vi "rethinkdb_launch.vi"(8 "error in (no error)":errorcluster, 9 "data_dir (\"\"=<appdir>\\rethinkdb_data)":path, 10 "http-port (5001)":u16=5001, 11 "rethinkdb.exe (\"\"=<appdir>\\rethinkdb.exe)":path) -> (0 "error out":errorcluster)   [LabVIEW 2017]
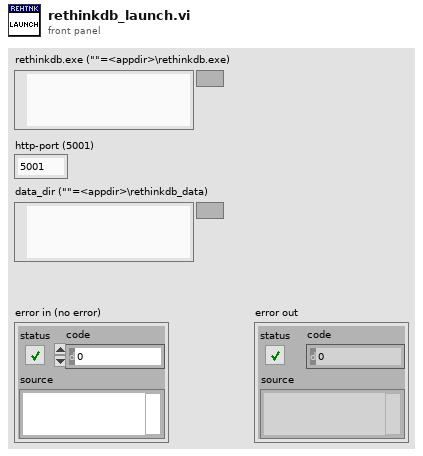
[diagram p1: front panel]
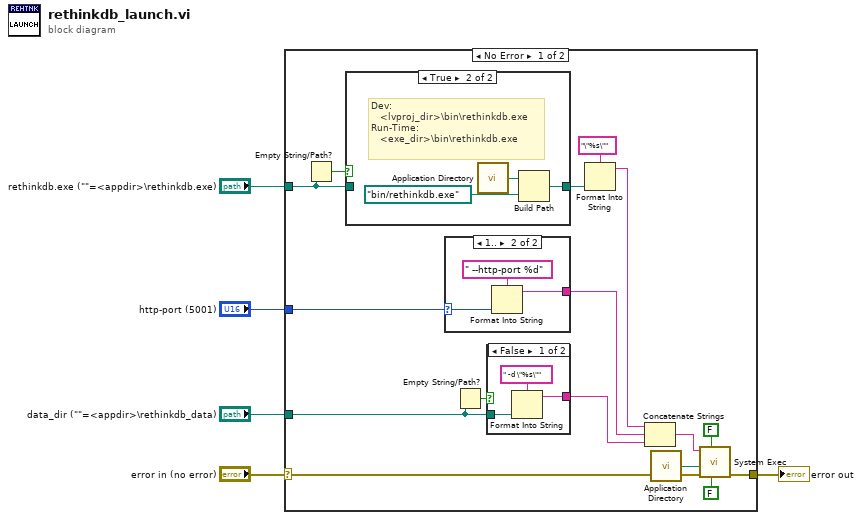
[diagram p0: block diagram]
diagram:
  n1 = case shown="No Error" "error in (no error)" {
    selector: "error in (no error)" -> [w21 w32]
    tunnel: [w20 w32] -> w4
    tunnel: "rethinkdb.exe (\"\"=<appdir>\\rethinkdb.exe)" -> [w16 _]
    tunnel: "http-port (5001)" -> [w14 _]
    tunnel: "data_dir (\"\"=<appdir>\\rethinkdb_data)" -> [w11 _]
    frame No Error {
      n2 = Empty String/Path?(string/path=w16) -> (empty?=w15:bool)
      n3 = case shown="True" w15 {
        tunnel: [w25 w27] -> w18
        tunnel: w16 -> [w25 _]
        frame False {
        }
        frame True {
          # "Dev:\n   <lvproj_dir>\\bin\\rethinkdb.exe\nRun-Time:\n   <exe_dir>\\bin\\rethinkdb.exe"
          n4 = call <vilib>:"Application Directory.vi"() -> ("Application Directory"=w28:path)
          n5 = Build Path(base path=w28, name or relative path=path "bin/rethinkdb.exe" ("Application Directory")) -> (appended path=w27:path)
        }
      }
      n6 = case shown="1.." w14 {
        selector: w14 -> [_ w24]
        tunnel: [_ w22] -> w12
        frame 0, Default {
        }
        frame 1.. {
          n7 = Format Into String(format string=" --http-port %d", w24) -> (resulting string=w22:string)  [unwired: 2 in, 1 out]
        }
      }
      n8 = Empty String/Path?(string/path=w11) -> (empty?=w10:bool)
      n9 = case shown="False" w10 {
        tunnel: w11 -> [w31 _]
        tunnel: [w29 _] -> w9
        frame False {
          n10 = Format Into String(format string=" -d \"%s\"", w31) -> (resulting string=w29:string)  [unwired: 2 in, 1 out]
        }
        frame True {
        }
      }
      n11 = Format Into String(format string="\"%s\"", w18) -> (resulting string=w13:string)  [unwired: 2 in, 1 out]
      n12 = Concatenate Strings(w13, w12, w9) -> (w8:string)
      n13 = call <vilib>:"Application Directory.vi"() -> ("Application Directory"=w19:path)
      n14 = call <vilib>:"System Exec.vi"("run minimized? (F)"=FALSE, "wait until completion? (T)"=FALSE, "error in (no error)"=w21, "working directory"=w19, "command line"=w8) -> ("error out"=w20:errorcluster)  [unwired: 3 in, 3 out]
    }
    frame Error {
    }
  }
  "error out" <- w4
